vi "Image Label.vi"() -> ()   [LabVIEW 2014]
doc: "This example shows how to label a binary image that contains multiple particles. The labeling process assigns a unique value to all the pixels that belong to a particle. Some processing functions in NI Vision require the input binary image to be labeled."
uses:
  <vilib>/vision/NI_Vision_Development_Module.lvlib
panel:
  out "Number of Particles Found":i32
  out "Extracted Image":T1(plugin-control) caption="Extracted Image (displayed using binary palette)"
  out "Image Source":T1(plugin-control)
  in  "Threshold Values":T2={"Minimum Value"=0.0, "Maximum Value"=150.0}
  in  "Connectivity":bool
  # "Overview: Demonstrates how to threshold an image, smooth the contours of the particles found using an Auto-Median morphological operator, and label the image.\nRequirements: NI Vision Development Module\nInstructions: Run the VI."
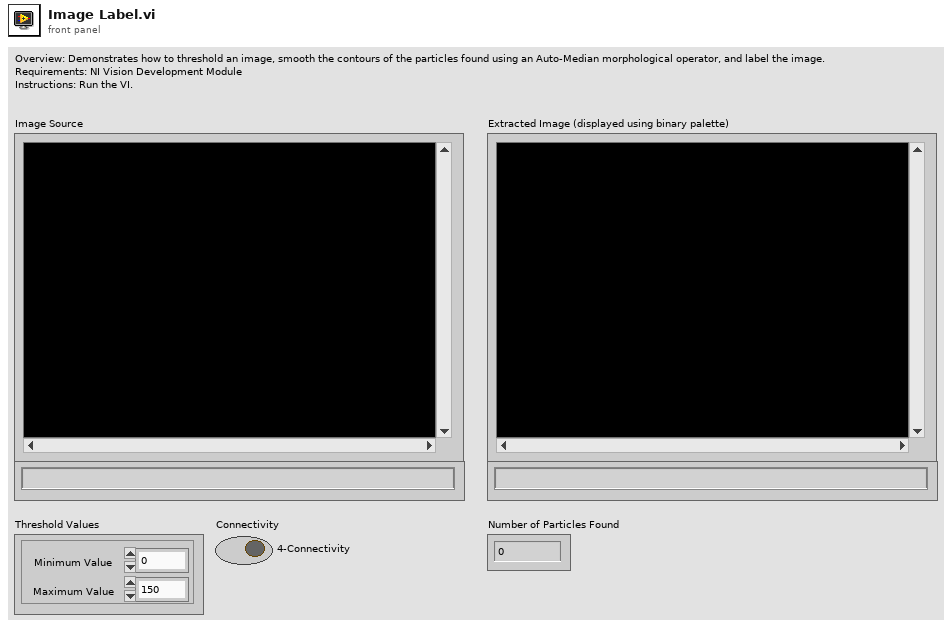
[diagram p1: front panel]
types:
  T1 = typedef "IMAQ Image.ctl" = refnum<image>
  T2 = cluster{"Minimum Value":sgl, "Maximum Value":sgl}
  T3 = enum32{"AutoM", "Close", "Dilate", "Erode", "Gradient", "Gradient out", "Gradient in", "Hit miss", "Open", "PClose", "POpen", "Thick", "Thin"}
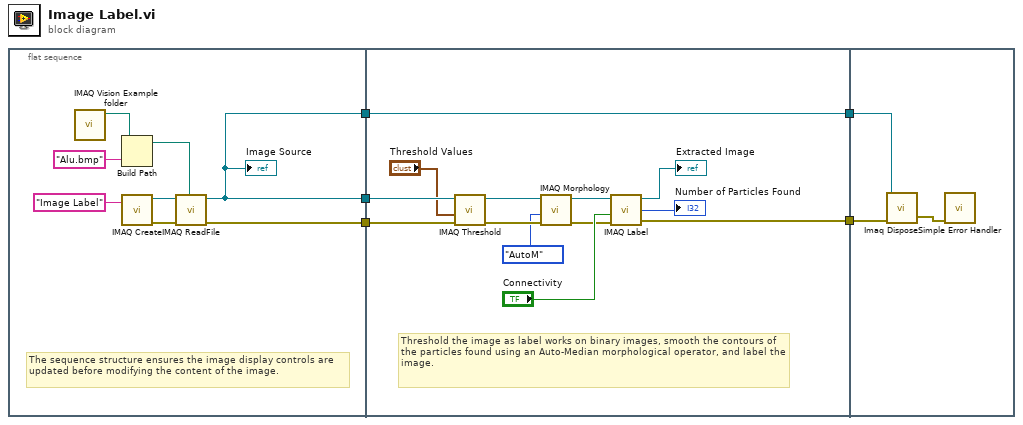
[diagram p0: block diagram]
diagram:
  n1 = flat-sequence {
    tunnel: [w7] -> w4
    tunnel: [w6] -> w3
    tunnel: [w6] -> w1
    tunnel: [w20] -> w5
    tunnel: w4 -> [w19]
    tunnel: w3 -> [w18]
    tunnel: [w17] -> w2
    tunnel: w1 -> [w17]
    tunnel: w5 -> [w29]
    tunnel: w2 -> [w27]
    frame #0 {
      # "The sequence structure ensures the image display controls are updated before modifying the content of the image."
      n2 = call "IMAQ Vision Example folder.vi"() -> ("Example Image Path"=w13:path)  [unwired: 11 in]
      n3 = Build Path(base path=w13, name or relative path="Alu.bmp") -> (appended path=w8:path)
      n4 = call "IMAQ Create"("Image Name"="Image Label") -> ("New Image"=w9:T1, "error out"=w10:errorcluster)  [unwired: 4 in]
      n5 = call "IMAQ ReadFile"("File Path"=w8, "error in (no error)"=w10, "Image"=w9) -> ("error out"=w7:errorcluster, "Image Out"=w6:T1)  [unwired: 4 in, 3 out]
      "Image Source" <- w6
    }
    frame #1 {
      # "Threshold the image as label works on binary images, smooth the contours of the particles found using an Auto-Median morphological operator, and label the image."
      n6 = call "IMAQ Threshold"("error in (no error)"=w19, "Range"="Threshold Values", "Image Src"=w18) -> ("error out"=w23:errorcluster, "Image Dst Out"=w26:T1)  [unwired: 7 in]
      n7 = call "IMAQ Morphology"("error in (no error)"=w23, "Operation"=T3."AutoM", "Image Src"=w26) -> ("error out"=w22:errorcluster, "Image Dst Out"=w24:T1)  [unwired: 7 in]
      n8 = call "IMAQ Label"("error in (no error)"=w22, "Connectivity 4/8 (8)"="Connectivity", "Image Src"=w24) -> ("error out"=w20:errorcluster, "Number of Particles"=→"Number of Particles Found":i32, "Image Dst Out"=→"Extracted Image":T1)  [unwired: 1 in]
    }
    frame #2 {
      n9 = call "Imaq Dispose"("Image"=w27, "error in (no error)"=w29) -> ("error out"=w28:errorcluster)  [unwired: 4 in]
      n10 = call <vilib>:"Simple Error Handler.vi"("error in (no error)"=w28) -> ()  [unwired: 4 in, 5 out]
    }
  }
